vi "Modbas TCP test.vi"   [LabVIEW 2019]
uses:
  <vilib>/NI/Modbus Library/API/Wrapper/Create TCP Master.vi
  <vilib>/NI/Modbus Library/API/Master/Modbus Master.lvclass
  <vilib>/NI/Modbus Library/API/Wrapper/API Main.lvlib
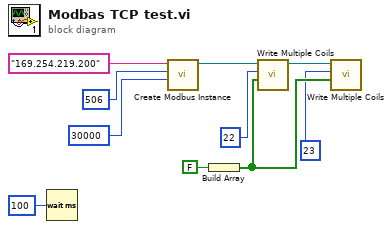
[diagram p0: block diagram]
diagram:
  n1 = Wait (ms)(milliseconds to wait=u32 100 ("等待时间（毫秒）")) -> ()  [unwired: 1 out]
  n2 = call-poly <vilib>:"Create Modbus Instance.vi"("connect timeout ms"=30000, "port (502)"=u16 506, "address"="169.254.219.200") -> ("TCP master instance"=w2:refnum<class "Modbus Master.lvclass">)  [unwired: 7 in, 1 out]
  n3 = Build Array(FALSE) -> (w4:bool[])
  n4 = call-dynamic "Write Multiple Coils.vi"("coils to write"=w4, "starting address"=u16 22, "Modbus master in"=w2) -> ("Modbus master out"=w5:refnum<class "Modbus Master.lvclass">)  [unwired: 7 in, 1 out]
  n5 = call-dynamic "Write Multiple Coils.vi"("coils to write"=w4, "starting address"=u16 23, "Modbus master in"=w5) -> ()  [unwired: 7 in, 2 out]
